vi "Rover_mv.vi"() -> ()   [LabVIEW 2018]
uses:
  <vilib>/Instr/_visa.llb/VISA Configure Serial Port (Instr).vi
  <vilib>/Utility/file.llb/Write Delimited Spreadsheet (string).vi
  <vilib>/Utility/inputDevices.llb/keyboardAcquire.vi
  <vilib>/sound2/lvsound2.llb/Sound File Read Open.vi
  <vilib>/Utility/inputDevices.llb/closeKeyboard.vi
  <resource>/objmgr/imaqdx.rc
  <vilib>/vision/driver/NI_Vision_Acquisition_Software.lvlib
  <vilib>/vision/NI_Vision_Development_Module.lvlib
panel:
  in  "path 5":path=path "C:/Users/向成/Desktop/ROVER PROJECT/LABVIEW codes/objet_detected.wav" caption="路径"
  in  "path 4":path=path "C:/Users/向成/Desktop/ROVER PROJECT/LABVIEW codes/objet_detected.wav" caption="路径"
  in  "Frames Per Second":u32=9
  in  "Camera port":refnum<k21>="cam5" caption="IMAQdx Session"
  out "Image 2":T1(plugin-control)
  out "postition x":dbl
  out "postition y":dbl
  in  "Video Modes":i32(listbox)
  out "DIS":dbl(knob) scale=0.0..500.0
  out "Right view":bool
  out "Left view":bool
  out "Front view":bool
  out "AIR":dbl(knob) scale=500.0..1300.0
  out "Air Pressure Monitoring":string
  in  "path 3":path=path "C:/Users/向成/Desktop/ROVER PROJECT/LABVIEW codes/voice recognition/danger.wav" caption="路径"
  out "Distance Monitoring":string
  in  "Sensors activation":bool
  out "TEM":dbl(slide) caption="量表" scale=0.0..50.0
  out "Temperature Monitoring":string
  out "gear":dbl(slide) scale=0.0..3.0
  out "LEFT":bool
  out "RIGHT":bool
  out "UP":bool
  out "DOWN":bool
  out "字符串监控":string
  in  "?":bool
  in  "Serial port":refnum<visa-resource-name>="COM4"
  # "Gear Stick Control"
  # "Motors Control"
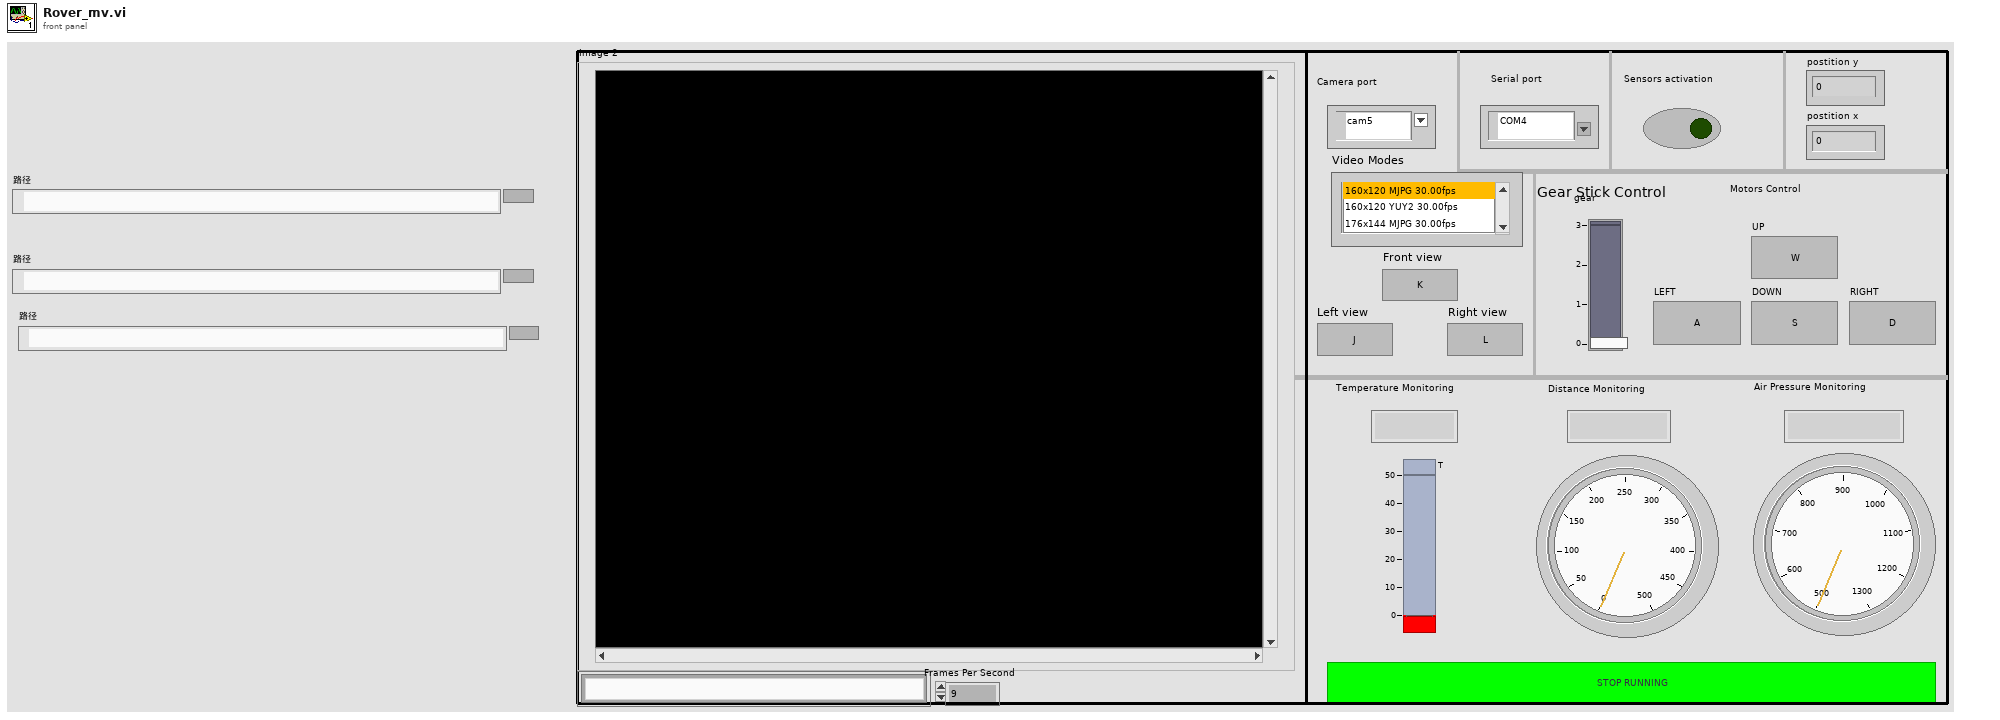
[diagram p1: front panel]
types:
  T1 = typedef "IMAQ Image.ctl" = refnum<image>
  T2 = enum16{"0", "1", "2", "3", "4", "5", "6", "7", "8", "9", "A", "B", "C", "D", "E", "F", "G", "H", "I", "J", "K", "L", "M", "N", "O", "P", "Q", "R", "S", "T", "U", "V", "W", "X", "Y", "Z", "F1", "F2", "F3", "F4", "F5", "F6", "F7", "F8", "F9", "F10", "F11", "F12", "F13", "F14", "F15", "ADD", "BACK", "BACKSLASH", "CAPITAL", "COMMA", "DECIMAL", "DELETE", "DIVIDE", "DOWN", "END", "EQUALS", "ESCAPE", "GRAVE (`)", "HOME", "INSERT", "LBRACKET", "LCONTROL", "LEFT", "L ALT", "LSHIFT", "LWIN", "MINUS", "MULTIPLY", "NEXT", "NUMLOCK", "NUMPAD_0", "NUMPAD_1", "NUMPAD_2", "NUMPAD_3", "NUMPAD_4", "NUMPAD_5", "NUMPAD_6", "NUMPAD_7", "NUMPAD_8", "NUMPAD_9", "PAUSE", "PERIOD", "PRIOR (PG UP)", "RBRACKET", "RCONTROL", "RETURN", "RIGHT", "R ALT", "RSHIFT", "RWIN", "SCROLL", "SEMICOLON", "SLASH", "SPACE", "SUBTRACT", "TAB", "UP", "ENTER (num pad)", "' (quote)"}
  T3 = typedef "Image Type" = u32
  T4 = typedef "IMAQdx.ctl" = refnum<k21>
  T5 = typedef "AviRefnum.ctl" = refnum<k1>
  T6 = enum16{"0", "1", "2", "3", "4", "5", "6", "7", "8", "9", "A", "B", "C", "D", "E", "F", "G", "H", "I", "J", "K", "L", "M", "N", "O", "P", "Q", "R", "S", "T", "U", "V", "W", "X", "Y", "Z", "F1", "F2", "F3", "F4", "F5", "F6", "F7", "F8", "F9", "F10", "F11", "F12", "F13", "F14", "F15", "ADD", "BACK", "BACKSLASH", "CAPITAL", "COMMA", "DECIMAL", "DELETE", "DIVIDE", "DOWN", "END", "EQUALS", "ESCAPE", "GRAVE (`)", "HOME", "INSERT", "LBRACKET", "LCONTROL", "LEFT", "L ALT", "LSHIFT", "LWIN", "MINUS", "MULTIPLY", "NEXT", "NUMLOCK", "NUMPAD_0", "NUMPAD_1", "NUMPAD_2", "NUMPAD_3", "NUMPAD_4", "NUMPAD_5", "NUMPAD_6", "NUMPAD_7", "NUMPAD_8", "NUMPAD_9", "PAUSE", "PERIOD", "PRIOR (PG UP)", "RBRACKET", "RCONTROL", "RETURN", "RIGHT", "R ALT", "RSHIFT", "RWIN", "SCROLL", "SEMICOLON", "SLASH", "SPACE", "SUBTRACT", "TAB", "UP", "ENTER (num pad)", "' (quote)"}[]
  T7 = typedef "Sound File Refnum.ctl" = refnum<file>
  T8 = typedef "IMAQ GM Match Report.ctl" = cluster{"Position":cluster{"x":sgl, "y":sgl}, "Angle":sgl, "Scale":sgl, "Score":sgl, "Bounding Box":cluster{"x":sgl, "y":sgl}[], "Contrast Reversed":bool, "Occlusion %":sgl, "Template Target Curve Score":sgl, "Target Template Curve Score":sgl, "Correlation Score":sgl}
  T9 = cluster{"Matches (Pattern Matching 1)[0]":T8, "Matches (Pattern Matching 1)[1]":T8, "Matches (Pattern Matching 1)[2]":T8, "Matches (Pattern Matching 1)[3]":T8}
  T10 = cluster{"Bounding Box[0]":cluster{"x":sgl, "y":sgl}, "Bounding Box[1]":cluster{"x":sgl, "y":sgl}, "Bounding Box[2]":cluster{"x":sgl, "y":sgl}, "Bounding Box[3]":cluster{"x":sgl, "y":sgl}}
  T11 = cluster{"[0]":sgl, "[1]":sgl, "[2]":sgl, "[3]":sgl}
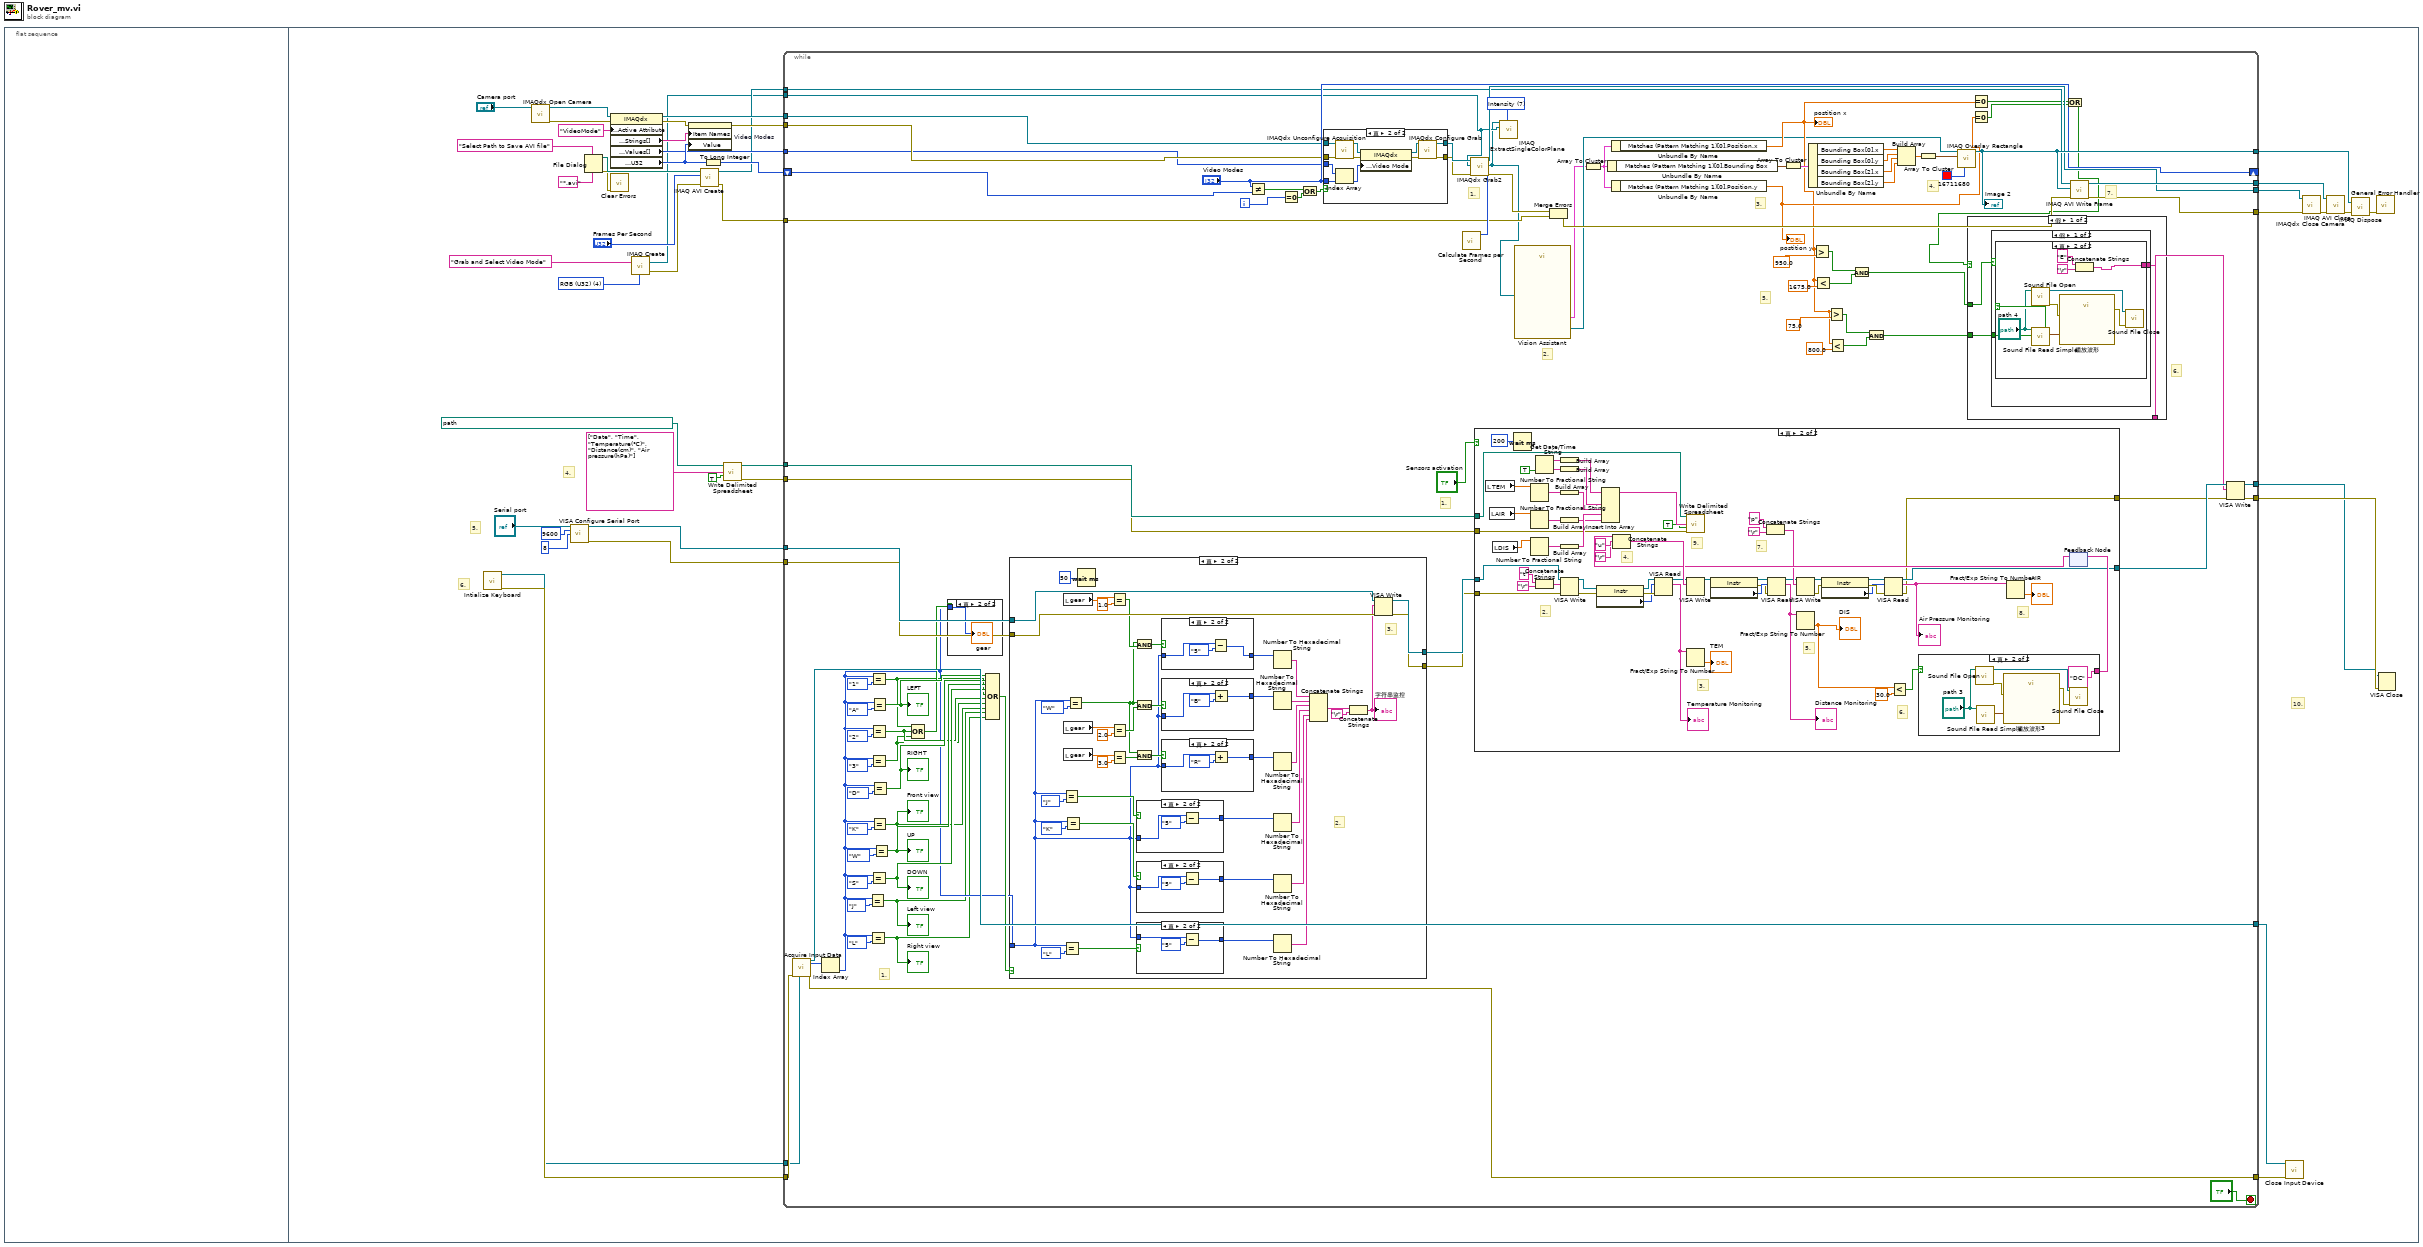
[diagram p0: block diagram]
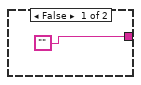
[diagram p2: hidden frame]
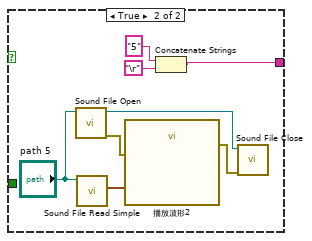
[diagram p3: hidden frame]
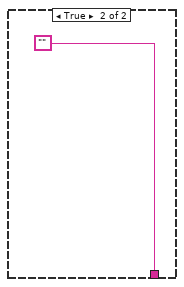
[diagram p4: hidden frame]
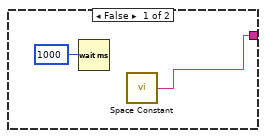
[diagram p7: hidden frame]
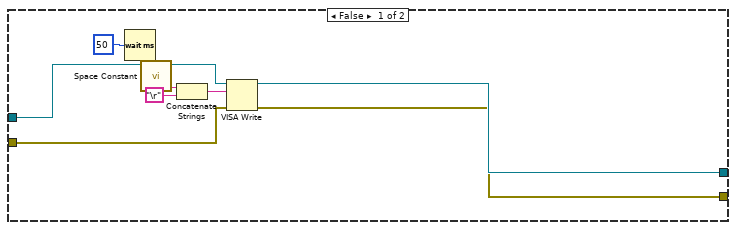
[diagram p9: hidden frame]
diagram:
  n1 = flat-sequence {
    frame #0 {
    }
    frame #1 {
      w24 = T3 4 items=["Grayscale (U8)", "Grayscale (I16)", "Grayscale (SGL)", "Complex (CSG)", "RGB (U32)", "HSL (U32)", "RGB (U64)", "Grayscale (U16)"] ("Image Type")
      # "10."
      # "6."
      # "5."
      # "4."
      n2 = call <vilib>:"Intialize Keyboard.vi"() -> ("error out"=w40:errorcluster, "device ID"=w39:refnum<k1>)  [unwired: 10 in]
      n3 = call <vilib>:"IMAQdx Open Camera.vi"("Session In"="Camera port") -> ("error out"=w19:errorcluster, "Session Out"=w18:T4)  [unwired: 2 in, 7 out]
      n4 = call-poly "VISA Configure Serial Port"("VISA resource name"="Serial port", "baud rate (9600)"=u32 9600, "data bits (8)"=u16 8) -> ("VISA resource name out"=w44:refnum<visa-resource-name>, "error out"=w45:errorcluster)  [unwired: 3 in, 8 out]
      n5 = File Dialog(6:"*.avi" ("pattern"), 7:"Select Path to Save AVI file" ("prompt")) -> (0:w13:errorcluster, 3:w14:path)  [unwired: 1 in, 6 out]
      n6 = property class="IMAQdx"(reference=w18, error in=w19, "Camera Attributes:Active Attribute"="VideoMode" ("ActiveAttribute")) -> (reference out=w7:T4, error out=w12:errorcluster, "Camera Attributes:Enum:Strings[]"=w11:string[], "Camera Attributes:Enum:Values[]"=w5:u32[], "Camera Attributes:Value:U32"=w10:u32)
      n7 = call <vilib>:"Clear Errors.vi"("error in (no error)"=w13) -> ()  [unwired: 5 in, 2 out]
      n8 = call "IMAQ Create"("Image Name"="Grab and Select Video Mode", "Image Type"=w24) -> ("New Image"=w3:T1, "error out"=w16:errorcluster)  [unwired: 2 in, 1 out]
      n9 = property on="Video Modes" class="LstBox (严格)"(error in=w12, "Item Names"=w11, "Value"=w10) -> (error out=w6:errorcluster)  [unwired: 1 in, 1 out]
      n10 = call "IMAQ AVI Create"("error in (no error)"=w16, "Frames Per Second"="Frames Per Second", "AVI Path"=w14) -> ("error out"=w8:errorcluster, "Avi Refnum"=w4:T5)  [unwired: 4 in, 3 out]
      n11 = To Long Integer(number=w10) -> (32bit integer=w9:i32)
      n12 = call-poly <vilib>:"Write Delimited Spreadsheet.vi"("file path (dialog if empty)"=path "C:/Users/向成/Desktop/rover_project/Data_Storage/data_acquired", "1D data"=string[] ["Date", "Time", "Temperature(℃)", "Distance(cm)", "Air pressure(hPa)"], "append to file? (new file:F)"=TRUE) -> ("new file path (Not A Path if cancelled)"=w33:path, "error out"=w32:errorcluster)  [unwired: 11 in]
      n13 = while {
        tunnel: w39 -> [w135]
        tunnel: w40 -> [w136]
        tunnel: w44 -> [w133]
        tunnel: w45 -> [w132]
        tunnel: [w134] -> w42
        tunnel: [w131] -> w43
        tunnel: w33 -> [w102]
        tunnel: w32 -> [w101]
        tunnel: [w100] -> w28
        tunnel: [w99] -> w27
        tunnel: [w98] -> w26
        tunnel: [w97] -> w25
        shift-right: ["Video Modes"] -> _
        shift-left: w9 -> [w76]
        tunnel: w8 -> [w74]
        tunnel: w7 -> [w73]
        tunnel: w6 -> [w72]
        tunnel: w5 -> [w71]
        tunnel: w4 -> [w70]
        tunnel: w3 -> [w69]
        tunnel: [w65] -> w2
        tunnel: [w64] -> w1
        i -> [w75]
        stop <- "?" stop-if-true
        w96 = 7 items=["Red", "Green", "Blue", "Hue", "Saturation", "Luminance", "Value", "Intensity"] ("Color Plane")
        # "7."
        # "6."
        # "5."
        # "4."
        # "3."
        # "2."
        # "1."
        # "1."
        # "1."
        n14 = call-poly <vilib>:"Acquire Input Data.vi"("device ID"=w135, "error in (no error)"=w136) -> ("device ID"=w134:refnum<k1>, "keys pressed"=w128:T6, "error out"=w131:errorcluster)  [unwired: 15 in]
        n15 = Index Array(array=w128) -> (element=w106:T2)  [unwired: 1 in]
        n16 = Equal?(x=w106, y=T2."J") -> (x = y?=w105:bool)
        "Left view" <- w105
        n17 = Equal?(x=w106, y=T2."L") -> (x = y?=w104:bool)
        "Right view" <- w104
        n18 = Equal?(x=w106, y=T2."1") -> (x = y?=w116:bool)
        n19 = Equal?(x=w106, y=T2."2") -> (x = y?=w115:bool)
        n20 = Equal?(x=w106, y=T2."3") -> (x = y?=w114:bool)
        n21 = Equal?(x=w106, y=T2."S") -> (x = y?=w118:bool)
        "DOWN" <- w118
        n22 = Equal?(x=w106, y=T2."A") -> (x = y?=w121:bool)
        "LEFT" <- w121
        n23 = Equal?(x=w106, y=T2."K") -> (x = y?=w109:bool)
        "Front view" <- w109
        n24 = Equal?(x=w106, y=T2."D") -> (x = y?=w120:bool)
        "RIGHT" <- w120
        n25 = Equal?(x=w106, y=T2."W") -> (x = y?=w119:bool)
        "UP" <- w119
        n26 = Compound Arithmetic op=OR ("复合运算")(w116, w115, w114) -> (w117:bool)
        n27 = case shown="真" w117 {
          tunnel: w106 -> [_ w241]
          frame False {
          }
          frame True {
            "gear" <- w241
          }
        }
        n28 = Compound Arithmetic op=OR ("复合运算")(w121, w120, w119, w118, w116, w115, w114, w109, w105, w104) -> (w127:bool)
        n29 = case shown="真" w127 {
          tunnel: [w244 w289] -> w113
          tunnel: [w243 w288] -> w112
          tunnel: w106 -> [_ w253]
          tunnel: w133 -> [w245 w287]
          tunnel: w132 -> [w246 w286]
          frame False {
            n30 = Wait (ms)(milliseconds to wait=u32 50 ("等待时间（毫秒）")) -> ()  [unwired: 1 out]
            n31 = call <vilib>:"Space Constant.vi"() -> ("String"=w247:string)
            n32 = Concatenate Strings(w247, "\r") -> (w249:string)
            n33 = VISA Write(VISA resource name=w245, write buffer=w249, error in (no error)=w246) -> (VISA resource name out=w244:refnum<visa-resource-name>, error out=w243:errorcluster)  [unwired: 1 out]
          }
          frame True {
            # "3."
            # "2."
            n34 = Equal?(x=w253, y=T2."J") -> (x = y?=w259:bool)
            n35 = Equal?(x=w253, y=T2."L") -> (x = y?=w257:bool)
            n36 = local read "gear"() -> (w284:dbl)
            n37 = local read "gear"() -> (w278:dbl)
            n38 = local read "gear"() -> (w273:dbl)
            n39 = Equal?(x=w253, y=T2."K") -> (x = y?=w258:bool)
            n40 = Equal?(x=w253, y=T2."W") -> (x = y?=w265:bool)
            n41 = Wait (ms)(milliseconds to wait=u32 50 ("等待时间（毫秒）")) -> ()  [unwired: 1 out]
            n42 = Equal?(x=w284, y=1.0) -> (x = y?=w282:bool)
            n43 = Equal?(x=w278, y=2.0) -> (x = y?=w276:bool)
            n44 = Equal?(x=w273, y=3.0) -> (x = y?=w274:bool)
            n45 = And(x=w265, y=w282) -> (x .and. y?=w281:bool)
            n46 = And(x=w265, y=w276) -> (x .and. y?=w280:bool)
            n47 = And(x=w265, y=w274) -> (x .and. y?=w266:bool)
            n48 = case shown="真" w259 {
              tunnel: [_ w298] -> w256
              tunnel: w253 -> [_ w297]
              frame False {
              }
              frame True {
                n49 = Subtract(x=w297, y=T2."5") -> (x-y=w298:u16)
              }
            }
            n50 = case shown="真" w258 {
              tunnel: [_ w295] -> w255
              tunnel: w253 -> [_ w294]
              frame False {
              }
              frame True {
                n51 = Subtract(x=w294, y=T2."5") -> (x-y=w295:u16)
              }
            }
            n52 = case shown="真" w257 {
              tunnel: [_ w292] -> w254
              tunnel: w253 -> [_ w291]
              frame False {
              }
              frame True {
                n53 = Subtract(x=w291, y=T2."5") -> (x-y=w292:u16)
              }
            }
            n54 = case shown="真" w281 {
              tunnel: w253 -> [w306 w309]
              tunnel: [w306 w307] -> w279
              frame False {
              }
              frame True {
                n55 = Subtract(x=w309, y=T2."5") -> (x-y=w307:u16)
              }
            }
            n56 = case shown="真" w280 {
              tunnel: [_ w304] -> w272
              tunnel: w253 -> [_ w303]
              frame False {
              }
              frame True {
                n57 = Add(x=w303, y=T2."B") -> (x+y=w304:u16)
              }
            }
            n58 = case shown="真" w266 {
              tunnel: [_ w301] -> w269
              tunnel: w253 -> [_ w300]
              frame False {
              }
              frame True {
                n59 = Add(x=w300, y=T2."R") -> (x+y=w301:u16)
              }
            }
            n60 = Number To Hexadecimal String(2:w279) -> (0:w270:string)  [unwired: 1 in]
            n61 = Number To Hexadecimal String(2:w272) -> (0:w271:string)  [unwired: 1 in]
            n62 = Number To Hexadecimal String(2:w269) -> (0:w268:string)  [unwired: 1 in]
            n63 = Number To Hexadecimal String(2:w256) -> (0:w252:string)  [unwired: 1 in]
            n64 = Number To Hexadecimal String(2:w255) -> (0:w250:string)  [unwired: 1 in]
            n65 = Number To Hexadecimal String(2:w254) -> (0:w251:string)  [unwired: 1 in]
            n66 = Concatenate Strings(w270, w271, w268, w252, w250, w251) -> (w267:string)
            n67 = Concatenate Strings(w267, "\r") -> (w264:string)
            "字符串监控" <- w264
            n68 = VISA Write(VISA resource name=w287, write buffer=w264, error in (no error)=w286) -> (VISA resource name out=w289:refnum<visa-resource-name>, error out=w288:errorcluster)  [unwired: 1 out]
          }
        }
        n69 = Not Equal?(x="Video Modes", y=w76) -> (x != y?=w83:bool)
        n70 = Equal To 0?(x=w75) -> (x = 0?=w82:bool)
        n71 = Or(x=w83, y=w82) -> (x .or. y?=w84:bool)
        n72 = case shown="真" w84 {
          tunnel: [w161 w169] -> w81
          tunnel: [w160 w170] -> w80
          tunnel: "Video Modes" -> [_ w172]
          tunnel: w71 -> [_ w165]
          tunnel: w73 -> [w161 w163]
          tunnel: w72 -> [w160 w162]
          frame False {
          }
          frame True {
            n73 = call <vilib>:"IMAQdx Unconfigure Acquisition.vi"("error in"=w162, "Session In"=w163) -> ("error out"=w166:errorcluster, "Session Out"=w171:T4)  [unwired: 8 out]
            n74 = Index Array(array=w165, index=w172) -> (element=w164:u32)
            n75 = property class="IMAQdx"(reference=w171, error in=w166, "Acquisition Attributes:Video Mode"=w164) -> (reference out=w168:T4, error out=w167:errorcluster)
            n76 = call <vilib>:"IMAQdx Configure Grab.vi"("error in"=w167, "Session In"=w168) -> ("error out"=w170:errorcluster, "Session Out"=w169:T4)  [unwired: 1 in, 7 out]
          }
        }
        n77 = call <vilib>:"IMAQdx Grab2.vi"("error in"=w80, "Image In"=w69, "Session In"=w81) -> ("error out"=w79:errorcluster, "Buffer Number Out"=w78:u32, "Image Out"=w46:T1, "Session Out"=w97:T4)  [unwired: 5 in]
        n78 = call <vilib>:"Calculate Frames per Second.vi"("Buffer Number"=w78) -> ()  [unwired: 8 in, 3 out]
        n79 = case shown="真" "Sensors activation" {
          tunnel: w113 -> [w174 w232]
          tunnel: w112 -> [w173 w231]
          tunnel: w102 -> [_ w216]
          tunnel: w101 -> [_ w214]
          tunnel: [w174 w178] -> w67
          tunnel: [w173 w175] -> w66
          frame False {
          }
          frame True {
            # "8."
            # "7."
            # "4."
            # "6."
            # "5."
            # "3."
            # "2."
            # "9."
            n80 = local read "TEM"() -> (w230:dbl)
            n81 = local read "AIR"() -> (w228:dbl)
            n82 = local read "DIS"() -> (w176:dbl)
            n83 = Wait (ms)(milliseconds to wait=u32 200 ("等待时间（毫秒）")) -> ()  [unwired: 1 out]
            n84 = Number To Fractional String(number=w230) -> (F-format string=w229:string)  [unwired: 3 in]
            n85 = Number To Fractional String(number=w228) -> (F-format string=w227:string)  [unwired: 3 in]
            n86 = Number To Fractional String(number=w176) -> (F-format string=w226:string)  [unwired: 3 in]
            n87 = Get Date/Time String(want seconds? (F)=TRUE ("需要秒？(F)")) -> (date string=w220:string, time string=w221:string)  [unwired: 2 in]
            n88 = Concatenate Strings("t" ("字符串"), "\r") -> (w208:string)
            n89 = Build Array(w220) -> (w222:string[])
            n90 = Build Array(w221) -> (w223:string[])
            n91 = Build Array(w229) -> (w225:string[])
            n92 = Build Array(w227) -> (w218:string[])
            n93 = Build Array(w226) -> (w219:string[])
            n94 = VISA Write(VISA resource name=w232, write buffer=w208, error in (no error)=w231) -> (VISA resource name out=w210:refnum<visa-resource-name>, error out=w209:errorcluster)  [unwired: 1 out]
            n95 = property class="Instr"(reference=w210, error in=w209) -> (reference out=w213:refnum<visa-resource-name>, error out=w212:errorcluster, "Serial Settings:Number of Bytes at Serial Port"=w211:u32)
            n96 = Insert Into Array(array=w222, new element #1=w223, new element #2=w225, new element #3=w219, new element #4=w218) -> (w224:string[])  [unwired: 1 in]
            n97 = VISA Read(VISA resource name=w213, byte count=w211, error in (no error)=w212) -> (VISA resource name out=w195:refnum<visa-resource-name>, read buffer=w203:string)  [unwired: 2 out]
            "Temperature Monitoring" <- w203
            n98 = call-poly <vilib>:"Write Delimited Spreadsheet.vi"("file path (dialog if empty)"=w216, "1D data"=w224, "append to file? (new file:F)"=TRUE, "error in (no error)"=w214) -> ()  [unwired: 10 in, 2 out]
            n99 = Fract/Exp String To Number(string=w203) -> (number=→"TEM":dbl)  [unwired: 3 in, 1 out]
            n100 = Concatenate Strings("p" ("字符串"), "\r") -> (w184:string)
            n101 = feedback #1() -> (w190:string)  [unwired: 1 in]
            n102 = Concatenate Strings(w190, "u" ("字符串"), "\r") -> (w200:string)
            n103 = VISA Write(VISA resource name=w195, write buffer=w200) -> (VISA resource name out=w196:refnum<visa-resource-name>)  [unwired: 1 in, 2 out]
            n104 = property class="Instr"(reference=w196) -> (reference out=w197:refnum<visa-resource-name>, error out=w198:errorcluster, "Serial Settings:Number of Bytes at Serial Port"=w199:u32)  [unwired: 1 in]
            n105 = VISA Read(VISA resource name=w197, byte count=w199, error in (no error)=w198) -> (VISA resource name out=w180:refnum<visa-resource-name>, read buffer=w191:string)  [unwired: 2 out]
            "Distance Monitoring" <- w191
            n106 = VISA Write(VISA resource name=w180, write buffer=w184) -> (VISA resource name out=w186:refnum<visa-resource-name>, error out=w185:errorcluster)  [unwired: 1 in, 1 out]
            n107 = Fract/Exp String To Number(string=w191) -> (number=w177:dbl)  [unwired: 3 in, 1 out]
            "DIS" <- w177
            n108 = property class="Instr"(reference=w186, error in=w185) -> (reference out=w189:refnum<visa-resource-name>, error out=w188:errorcluster, "Serial Settings:Number of Bytes at Serial Port"=w187:u32)
            n109 = VISA Read(VISA resource name=w189, byte count=w187, error in (no error)=w188) -> (VISA resource name out=w178:refnum<visa-resource-name>, read buffer=w179:string, error out=w175:errorcluster)  [unwired: 1 out]
            "Air Pressure Monitoring" <- w179
            n110 = Less?(x=w177, y=30.0) -> (x < y?=w194:bool)
            n111 = case shown="真" w194 {
              tunnel: [w233 "DC" ("字符串")] -> w192
              frame False {
                n112 = Wait (ms)(milliseconds to wait=u32 1000 ("等待时间（毫秒）")) -> ()  [unwired: 1 out]
                n113 = call <vilib>:"Space Constant.vi"() -> ("String"=w233:string)
              }
              frame True {
                n114 = call-poly <vilib>:"Sound File Open.vi"("path"="path 3") -> ("error out"=w237:errorcluster, "sound file refnum"=w235:T7)  [unwired: 9 in]
                n115 = call <vilib>:"Sound File Read Simple.vi"("path"="path 3") -> ("data"=w236:waveform(dbl)[])  [unwired: 7 in, 3 out]
                n116 = call "播放波形3"("Data"=w236, "error in"=w237) -> ("error out"=w238:errorcluster)  [unwired: 17 in]
                n117 = call <vilib>:"Sound File Close.vi"("error in (no error)"=w238, "sound file refnum"=w235) -> ()  [unwired: 9 in, 1 out]
              }
            }
            n118 = Fract/Exp String To Number(string=w179) -> (number=→"AIR":dbl)  [unwired: 3 in, 1 out]
            n119 = feedback-in #1(w192) -> ()
          }
        }
        n120 = call "IMAQ ExtractSingleColorPlane"("Color Plane"=w96, "Image Dst"=w69, "Image Src"=w46) -> ()  [unwired: 7 in, 2 out]
        n121 = call "Vision Assistant"("Image In"=w46) -> ("Image Out"=w48:T1, "Matches (Pattern Matching 1)"=w47:T8[])  [unwired: 24 in, 1 out]
        n122 = Merge Errors(w79, w74) -> (w85:errorcluster)
        n123 = Array To Cluster(array=w47) -> (cluster=w87:T9)
        n124 = Unbundle By Name(w87) -> ("Matches (Pattern Matching 1)[0].Bounding Box"=w95:cluster{"x":sgl, "y":sgl}[])
        n125 = Unbundle By Name(w87) -> ("Matches (Pattern Matching 1)[0].Position.x"=w50:sgl)
        "postition x" <- w50
        n126 = Unbundle By Name(w87) -> ("Matches (Pattern Matching 1)[0].Position.y"=w63:sgl)
        "postition y" <- w63
        n127 = Array To Cluster(array=w95) -> (cluster=w94:T10)
        n128 = Unbundle By Name(w94) -> ("Bounding Box[0].x"=w93:sgl, "Bounding Box[0].y"=w92:sgl, "Bounding Box[2].x"=w91:sgl, "Bounding Box[2].y"=w90:sgl)
        n129 = Greater?(x=w50, y=950.0) -> (0:w57:bool)
        n130 = Less?(x=w50, y=sgl 1675.0) -> (x < y?=w56:bool)
        n131 = Greater?(x=w50, y=75.0) -> (0:w52:bool)
        n132 = Less?(x=w50, y=sgl 800.0) -> (x < y?=w51:bool)
        n133 = And(x=w57, y=w56) -> (x .and. y?=w55:bool)
        n134 = And(x=w52, y=w51) -> (x .and. y?=w49:bool)
        n135 = Build Array(w93, w92, w91, w90) -> (w89:sgl[])
        n136 = Array To Cluster(array=w89) -> (cluster=w88:T11)
        n137 = call "IMAQ Overlay Rectangle"("Color"=u32 16711680, "Rectangle"=w88, "Image"=w48) -> ("Image Out"=w99:T1)  [unwired: 7 in, 1 out]
        "Image 2" <- w99
        n138 = Equal To 0?(x=w50) -> (x = 0?=w62:bool)
        n139 = Equal To 0?(x=w63) -> (x = 0?=w61:bool)
        n140 = Or(x=w62, y=w61) -> (x .or. y?=w59:bool)
        n141 = case shown="假" w59 {
          tunnel: [w139 ""] -> w60
          tunnel: w55 -> [w138 _]
          tunnel: w49 -> [w137 _]
          frame False {
            n142 = case shown="假" w138 {
              tunnel: [w141 w156] -> w139
              tunnel: w137 -> [w140 _]
              frame False {
                n143 = case shown="真" w140 {
                  tunnel: ["" w148] -> w141
                  frame False {
                  }
                  frame True {
                    n144 = call-poly <vilib>:"Sound File Open.vi"("path"="path 4") -> ("error out"=w145:errorcluster, "sound file refnum"=w143:T7)  [unwired: 9 in]
                    n145 = call <vilib>:"Sound File Read Simple.vi"("path"="path 4") -> ("data"=w144:waveform(dbl)[])  [unwired: 7 in, 3 out]
                    n146 = call "播放波形"("Data"=w144, "error in"=w145) -> ("error out"=w146:errorcluster)  [unwired: 17 in]
                    n147 = Concatenate Strings("E" ("字符串"), "\r") -> (w148:string)
                    n148 = call <vilib>:"Sound File Close.vi"("error in (no error)"=w146, "sound file refnum"=w143) -> ()  [unwired: 9 in, 1 out]
                  }
                }
              }
              frame True {
                n149 = call-poly <vilib>:"Sound File Open.vi"("path"="path 5") -> ("error out"=w153:errorcluster, "sound file refnum"=w151:T7)  [unwired: 9 in]
                n150 = call <vilib>:"Sound File Read Simple.vi"("path"="path 5") -> ("data"=w152:waveform(dbl)[])  [unwired: 7 in, 3 out]
                n151 = call "播放波形2"("Data"=w152, "error in"=w153) -> ("error out"=w154:errorcluster)  [unwired: 17 in]
                n152 = Concatenate Strings("5" ("字符串"), "\r") -> (w156:string)
                n153 = call <vilib>:"Sound File Close.vi"("error in (no error)"=w154, "sound file refnum"=w151) -> ()  [unwired: 9 in, 1 out]
              }
            }
          }
          frame True {
          }
        }
        n154 = call "IMAQ AVI Write Frame"("error in (no error)"=w85, "Image"=w99, "Avi Refnum"=w70) -> ("error out"=w98:errorcluster, "Avi Refnum (duplicate)"=w100:T5)  [unwired: 1 in, 6 out]
        n155 = VISA Write(VISA resource name=w67, write buffer=w60, error in (no error)=w66) -> (VISA resource name out=w64:refnum<visa-resource-name>, error out=w65:errorcluster)  [unwired: 1 out]
      }
      n156 = call-poly <vilib>:"Close Input Device.vi"("error in (no error)"=w43, "device ID"=w42) -> ()  [unwired: 8 in, 1 out]
      n157 = call <vilib>:"IMAQdx Close Camera.vi"("error in"=w26, "Session In"=w25) -> ("error out"=w30:errorcluster)  [unwired: 9 out]
      n158 = call "IMAQ AVI Close"("error in (no error)"=w30, "Avi Refnum"=w28) -> ("error out"=w29:errorcluster)  [unwired: 9 out]
      n159 = call "IMAQ Dispose"("Image"=w27, "error in (no error)"=w29) -> ("error out"=w31:errorcluster)  [unwired: 4 in]
      n160 = call <vilib>:"General Error Handler.vi"("error in (no error)"=w31) -> ()  [unwired: 2 in, 13 out]
      n161 = VISA Close(VISA resource name=w1, error in (no error)=w2) -> ()  [unwired: 1 out]
    }
  }
